vi "get_component_paths.vi"(8 "error in (no error)":errorcluster, 11 "GenericComponent in":refnum<class "GenericComponent.lvclass">) -> (0 "error out":errorcluster, 1 "component class path":path, 2 "specific component directory":path, 3 "GenericComponent out":refnum<class "GenericComponent.lvclass">, 5 "component type directory":path, 7 "components directory":path)   [LabVIEW 2011, in "GenericComponent.lvclass"]
uses:
  GenericComponent.lvclass
  xcontrols/XUserDropdown/XUserDropdown/XUserDropdown.xctl
panel:
  # "(e.g., C:\\helioscan\\components\\Stage\\StageDL090602SutterMP285\\StageDL090602SutterMP285\\StageDL090602SutterMP285.lvclass)"
  # "(e.g., C:\\helioscan\\components\\Stage\\StageDL090602SutterMP285\\StageDL090602SutterMP285\\)"
  # "(e.g., C:\\helioscan\\components\\Stage)"
  # "(e.g., C:\\helioscan\\components)"
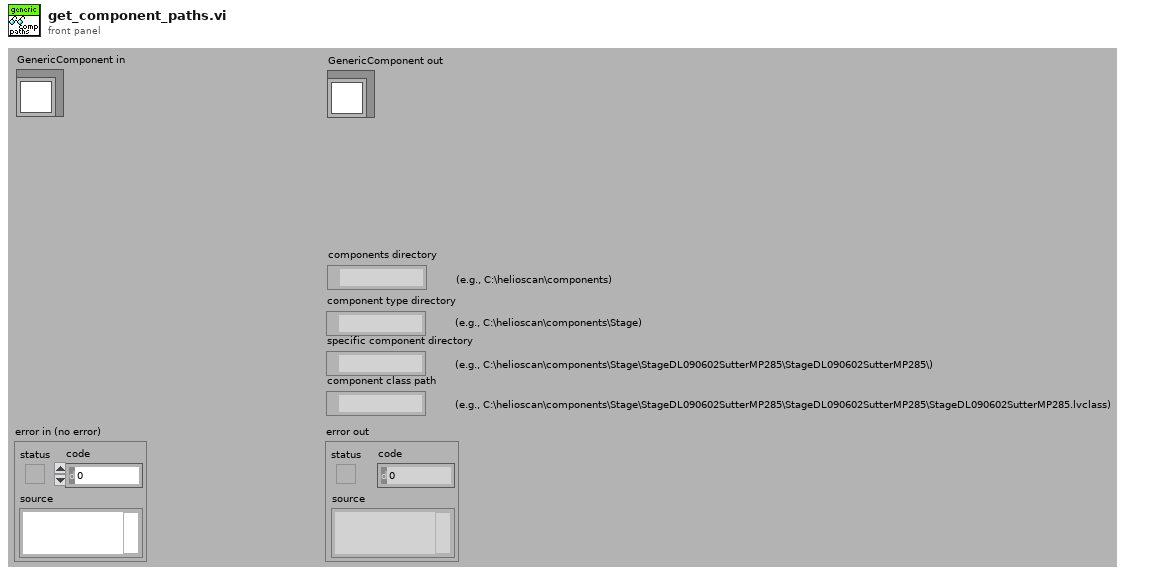
[diagram p1: front panel]
types:
  T1 = typedef "component_path_clusters.ctl" = cluster{"components directory":path, "component type directory":path, "specific component directory":path, "component class path":path}
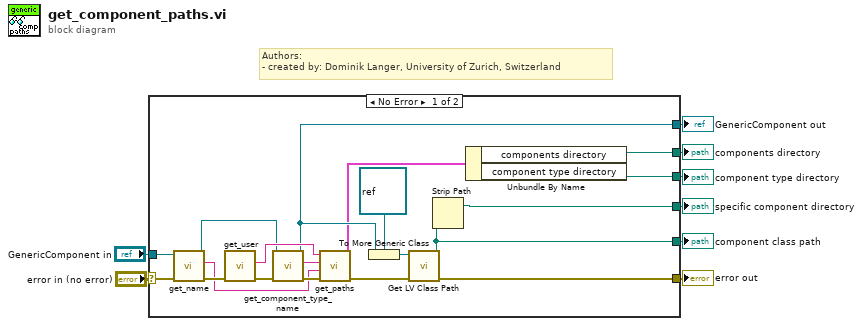
[diagram p0: block diagram]
diagram:
  # "Authors: \n- created by: Dominik Langer, University of Zurich, Switzerland"
  n1 = case shown="No Error" "error in (no error)" {
    selector: "error in (no error)" -> [w18 w29]
    tunnel: [w16 w29] -> w7
    tunnel: [w15 w28] -> w5
    tunnel: "GenericComponent in" -> [w17 w28]
    tunnel: [w14 _] -> w4
    tunnel: [w11 _] -> w3
    tunnel: [w10 _] -> w2
    tunnel: [w13 _] -> w1
    frame No Error {
      n2 = call-dynamic "get_name.vi"("error in (no error)"=w18, "GenericPlugin in"=w17) -> ("error out"=w20:errorcluster, "component name"=w19:string, "GenericPlugin out"=w9:refnum<class "GenericComponent.lvclass">)  [unwired: 7 in]
      n3 = call "get_user.vi"("error in (no error)"=w20) -> ("error out"=w22:errorcluster, "username out"=w23:string)  [unwired: 9 in]
      n4 = call-dynamic "get_component_type_name.vi"("error in (no error)"=w22, "GenericPlugin in"=w9) -> ("error out"=w25:errorcluster, "component type"=w24:string, "GenericPlugin out"=w15:refnum<class "GenericComponent.lvclass">)  [unwired: 7 in]
      n5 = call "get_paths.vi"("error in (no error)"=w25, "component name"=w19, "component type"=w24, "user"=w23) -> ("error out"=w21:errorcluster, "component paths"=w12:T1)  [unwired: 4 in, 2 out]
      n6 = To More Generic Class(target class=refnum<class> refnum ("LabVIEW Object"), reference=w15) -> (generic class reference=w27:refnum<class>)
      n7 = call <vilib>:"Get LV Class Path.vi"("error in (no error)"=w21, "object"=w27) -> ("error out"=w16:errorcluster, "class path"=w13:path)  [unwired: 8 in]
      n8 = Strip Path(path=w13) -> (stripped path=w14:path)  [unwired: 1 out]
      n9 = Unbundle By Name(w12) -> ("components directory"=w11:path, "component type directory"=w10:path)
    }
    frame Error {
    }
  }
  "error out" <- w7
  "GenericComponent out" <- w5
  "components directory" <- w3
  "component type directory" <- w2
  "specific component directory" <- w4
  "component class path" <- w1
